vi "2-3.vi"() -> ()   [LabVIEW 2016, in "Project.lvrbt"]
uses:
  Project.lvrbt
  <vilib>/NXT/Block Support/NXT_InputPort.ctl
  <vilib>/NXT/Block Support/NXT_OutputPort.ctl
  <vilib>/NXT/Dual Mode Library/Display/drawText_Center.vi
  <vilib>/NXT/NXTIO Xnodes/NXTIONodeSubVIs/NXTMoveMotors.vi
  <vilib>/NXT/Dual Mode Library/Waits/Wait_Num.vi
  <vilib>/NXT/NXTIO Xnodes/NXTIONodeSubVIs/LEGOStopAllMotors.vi
  <vilib>/NXT/Dual Mode Library/Sensors/EV3_Color_Reflect.vi
  <vilib>/NXT/Dual Mode Library/Sensors/EV3_Ultrasonic_CM.vi
  <vilib>/NXT/Dual Mode Library/Display/drawText.vi
  <vilib>/NXT/Dual Mode Library/Waits/Wait_LetGo.vi
  <vilib>/NXT/Dual Mode Library/Waits/Wait_Bump.vi
  <vilib>/NXT/Dual Mode Library/Sensors/Touch_Pressed.vi
  <vilib>/NXT/NXTIO Xnodes/AddressXNode/NXTIOAddress.xnode
  <vilib>/NXT/NXTIO Xnodes/NXTIOXNode/NXTIO.xnode
  <vilib>/NXT/Subs/LVHSConnector.ctl
  <vilib>/NXT/LegoClasses/BrickReference/BrickReference.lvclass
panel:
  in  "Stopp":bool
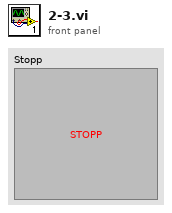
[diagram p1: front panel]
types:
  T1 = typedef "NXT_InputPort.ctl" = u32
  T2 = typedef "LVHSConnector.ctl" = refnum<class "BrickReference.lvclass">
  T3 = typedef "NXT_OutputPort.ctl" = u8
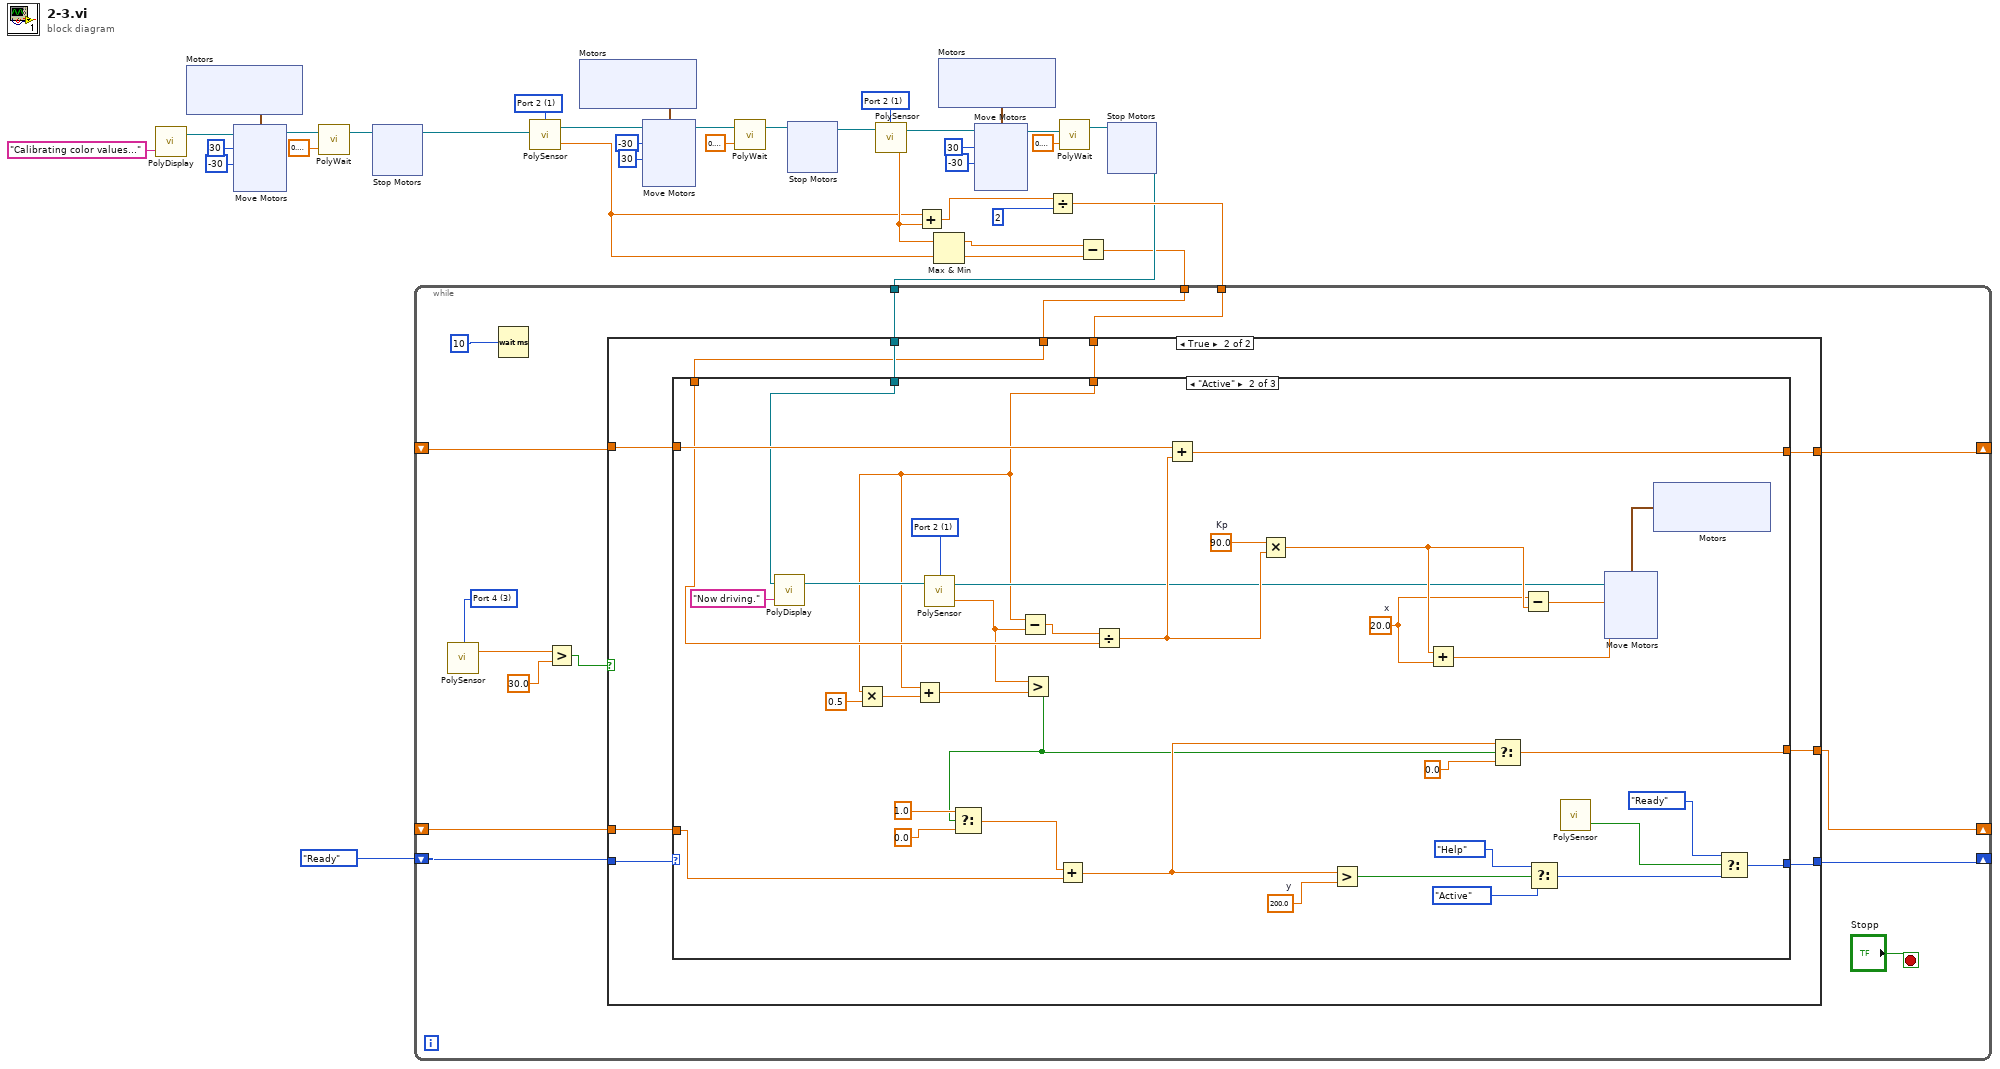
[diagram p0: block diagram]
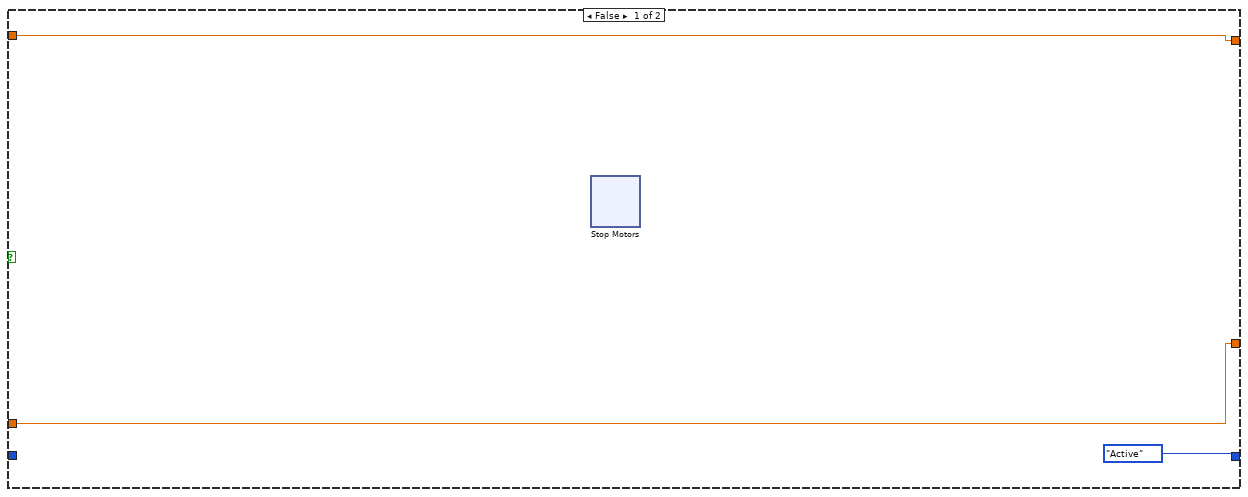
[diagram p2: hidden frame]
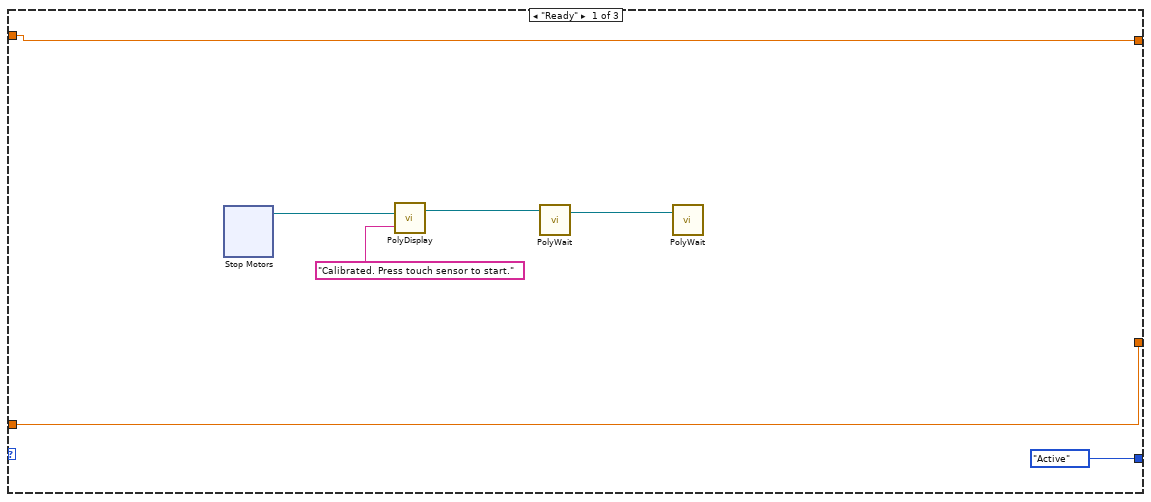
[diagram p3: hidden frame]
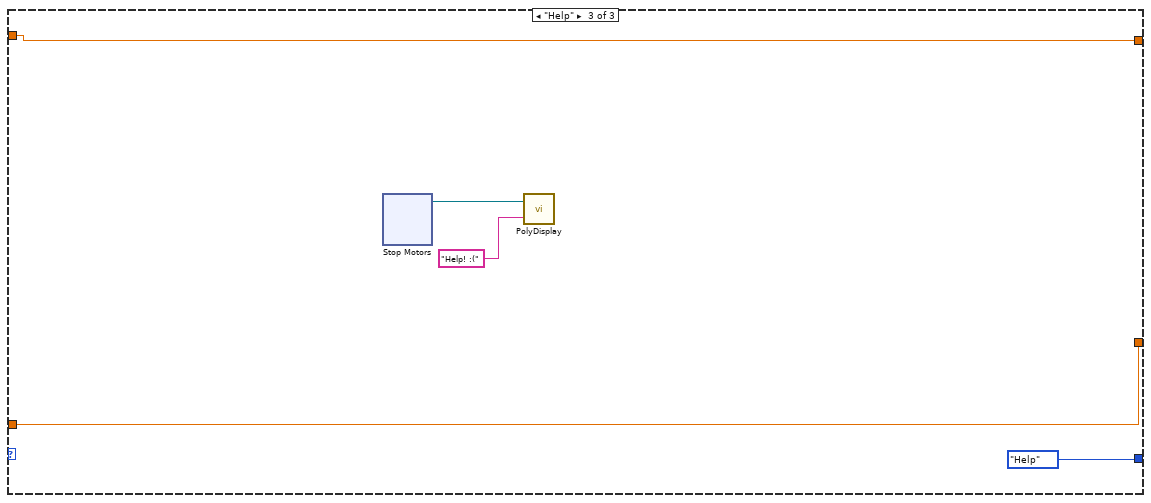
[diagram p4: hidden frame]
diagram:
  w30 = T1 1 items=["Port 1", "Port 2", "Port 3", "Port 4"] ("Port (Port 1)")
  w36 = T1 1 items=["Port 1", "Port 2", "Port 3", "Port 4"] ("Port (Port 1)")
  n1 = call-poly <vilib>:"PolyDisplay.vi"("Text"="Calibrating color values...") -> ("NXT/EV3"=w2:T2)  [unwired: 3 in]
  n2 = xnode "Motors"() -> ("Motor"=w34:cluster{"Port":T3, "Port":T3})
  n3 = xnode "Move Motors"("Power/Speed 2"=i8 -30, "Power/Speed 1"=i8 30, "Motors"=w34, "NXT/EV3"=w2) -> ("NXT/EV3"=w29:T2)
  n4 = call-poly <vilib>:"PolyWait.vi"("Time (1 sec)"=sgl 0.2, "NXT/EV3"=w29) -> ("NXT/EV3"=w25:T2)  [unwired: 2 in]
  n5 = xnode "Stop Motors"("NXT/EV3"=w25) -> ("NXT/EV3"=w24:T2)  [unwired: 1 in]
  n6 = call-poly <vilib>:"PolySensor.vi"("NXT/EV3"=w24, "Port (Port 1)"=w36) -> ("Scaled Value"=w1:sgl, "NXT/EV3"=w35:T2)  [unwired: 1 in]
  n7 = xnode "Motors"() -> ("Motor"=w33:cluster{"Port":T3, "Port":T3})
  n8 = xnode "Move Motors"("Power/Speed 2"=i8 30, "Power/Speed 1"=i8 -30, "Motors"=w33, "NXT/EV3"=w35) -> ("NXT/EV3"=w26:T2)
  n9 = call-poly <vilib>:"PolyWait.vi"("Time (1 sec)"=sgl 0.4, "NXT/EV3"=w26) -> ("NXT/EV3"=w23:T2)  [unwired: 2 in]
  n10 = xnode "Stop Motors"("NXT/EV3"=w23) -> ("NXT/EV3"=w22:T2)  [unwired: 1 in]
  n11 = call-poly <vilib>:"PolySensor.vi"("NXT/EV3"=w22, "Port (Port 1)"=w30) -> ("Scaled Value"=w9:sgl, "NXT/EV3"=w16:T2)  [unwired: 1 in]
  n12 = Add(x=w1, y=w9) -> (x+y=w12:sgl)
  n13 = Max & Min(x=w9, y=w1) -> (max(x,y)=w7:sgl, min(x,y)=w6:sgl)
  n14 = xnode "Motors"() -> ("Motor"=w19:cluster{"Port":T3, "Port":T3})
  n15 = xnode "Move Motors"("Power/Speed 2"=i8 -30, "Power/Speed 1"=i8 30, "Motors"=w19, "NXT/EV3"=w16) -> ("NXT/EV3"=w13:T2)
  n16 = Divide(x=w12, y=i16 2) -> (x/y=w10:sgl)
  n17 = call-poly <vilib>:"PolyWait.vi"("Time (1 sec)"=sgl 0.2, "NXT/EV3"=w13) -> ("NXT/EV3"=w14:T2)  [unwired: 2 in]
  n18 = Subtract(x=w7, y=w6) -> (x-y=w5:sgl)
  n19 = xnode "Stop Motors"("NXT/EV3"=w14) -> ("NXT/EV3"=w8:T2)  [unwired: 1 in]
  n20 = while {
    tunnel: w10 -> [w50]
    tunnel: w8 -> [w49]
    shift-right: [w47] -> _
    shift-left: _ -> [w48]
    tunnel: w5 -> [w37]
    shift-right: [w43] -> _
    shift-left: enum16{"Help", "Active", "Ready"}."Ready" -> [w46]
    shift-right: [w44] -> _
    shift-left: _ -> [w45]
    stop <- "Stopp" stop-if-true
    w40 = T1 3 items=["Port 1", "Port 2", "Port 3", "Port 4"] ("Port (Port 1)")
    n21 = call-poly <vilib>:"PolySensor.vi"("Port (Port 1)"=w40) -> ("Centimeters"=w42:sgl)  [unwired: 2 in, 1 out]
    n22 = Wait (ms) ("Warten (ms)")(milliseconds to wait=10) -> ()  [unwired: 1 out]
    n23 = Greater?(x=w42, y=sgl 30.0) -> (0:w39:bool)
    n24 = case shown="True" w39 {
      tunnel: w50 -> [_ w66]
      tunnel: w49 -> [_ w65]
      tunnel: w48 -> [w52 w64]
      tunnel: [w52 w63] -> w47
      tunnel: w37 -> [_ w62]
      tunnel: w46 -> [_ w61]
      tunnel: w45 -> [w53 w60]
      tunnel: [w53 w59] -> w44
      tunnel: [enum16{"Help", "Active", "Ready"}."Active" w58] -> w43
      frame False {
        n25 = xnode "Stop Motors"() -> ()  [unwired: 2 in, 1 out]
      }
      frame True {
        n26 = case "Case-Struktur" shown="\"Active\"" w61 {
          tunnel: w66 -> [_ w80 _]
          tunnel: w65 -> [_ w92 _]
          tunnel: w64 -> [w70 w107 w124]
          tunnel: [w70 w106 w124] -> w63
          tunnel: w62 -> [_ w105 _]
          tunnel: [enum16{"Help", "Active", "Ready"}."Active" w89 enum16{"Help", "Active", "Ready"}."Help"] -> w58
          tunnel: w60 -> [w69 w104 w125]
          tunnel: [w69 w94 w125] -> w59
          frame "Ready" {
            n27 = xnode "Stop Motors"() -> ("NXT/EV3"=w67:T2)  [unwired: 2 in]
            n28 = call-poly <vilib>:"PolyDisplay.vi"("Text"="Calibrated. Press touch sensor to start.", "NXT/EV3"=w67) -> ("NXT/EV3"=w71:T2)  [unwired: 2 in]
            n29 = call-poly <vilib>:"PolyWait.vi"("NXT/EV3"=w71) -> ("NXTEV3"=w68:T2)  [unwired: 3 in]
            n30 = call-poly <vilib>:"PolyWait.vi"("NXT/EV3"=w68) -> ()  [unwired: 3 in, 1 out]
          }
          frame "Active" {
            w103 = 200.0  # y
            w110 = sgl 90.0  # Kp
            w108 = 20.0  # x
            w112 = T1 1 items=["Port 1", "Port 2", "Port 3", "Port 4"] ("Port (Port 1)")
            n31 = call-poly <vilib>:"PolyDisplay.vi"("Text"="Now driving.", "NXT/EV3"=w92) -> ("NXT/EV3"=w86:T2)  [unwired: 2 in]
            n32 = Multiply(x=w80, y=0.5) -> (x*y=w81:dbl)
            n33 = Add(x=w80, y=w81) -> (x+y=w79:dbl)
            n34 = call-poly <vilib>:"PolySensor.vi"("NXT/EV3"=w86, "Port (Port 1)"=w112) -> ("Scaled Value"=w78:sgl, "NXT/EV3"=w88:T2)  [unwired: 1 in]
            n35 = Subtract(x=w80, y=w78) -> (x-y=w111:sgl)
            n36 = Greater?(x=w78, y=w79) -> (0:w82:bool)
            n37 = Select(t=1.0 ("x"), s=w82, f=0.0) -> (s? t:f=w99:dbl)
            n38 = Add(x=w99, y=w104) -> (x+y=w83:dbl)
            n39 = Divide(x=w111, y=w105) -> (x/y=w102:sgl)
            n40 = Add(x=w107, y=w102) -> (x+y=w106:sgl)
            n41 = Multiply(x=w110, y=w102) -> (x*y=w109:sgl)
            n42 = Greater?(x=w83, y=w103) -> (0:w98:bool)
            n43 = Add(x=w109, y=w108) -> (x+y=w84:dbl)
            n44 = Select(t=w83, s=w82, f=0.0) -> (s? t:f=w94:dbl)
            n45 = Subtract(x=w108, y=w109) -> (x-y=w85:dbl)
            n46 = Select(t=enum16{"Help", "Active", "Ready"}."Help", s=w98, f=enum16{"Help", "Active", "Ready"}."Active") -> (s? t:f=w90:enum16{"Help", "Active", "Ready"})
            n47 = call-poly <vilib>:"PolySensor.vi"() -> ("Yes / No"=w87:bool)  [unwired: 3 in, 1 out]
            n48 = xnode "Motors"() -> ("Motor"=w113:cluster{"Port":T3, "Port":T3})
            n49 = xnode "Move Motors"("Power/Speed 2"=w84, "Power/Speed 1"=w85, "Motors"=w113, "NXT/EV3"=w88) -> ()  [unwired: 1 out]
            n50 = Select(t=enum16{"Help", "Active", "Ready"}."Ready", s=w87, f=w90) -> (s? t:f=w89:enum16{"Help", "Active", "Ready"})
          }
          frame "Help" {
            n51 = xnode "Stop Motors"() -> ("NXT/EV3"=w126:T2)  [unwired: 2 in]
            n52 = call-poly <vilib>:"PolyDisplay.vi"("Text"="Help! :(", "NXT/EV3"=w126) -> ()  [unwired: 2 in, 1 out]
          }
        }
      }
    }
  }
